vi "DHE_DO_INIT.vi"(8 "error in":errorcluster) -> (0 "error out":errorcluster, 2 "response":string)   [LabVIEW 2016]
uses:
  SDSU_GBLVariables.vi
panel:
  out "ControllerConfigCluster":T1
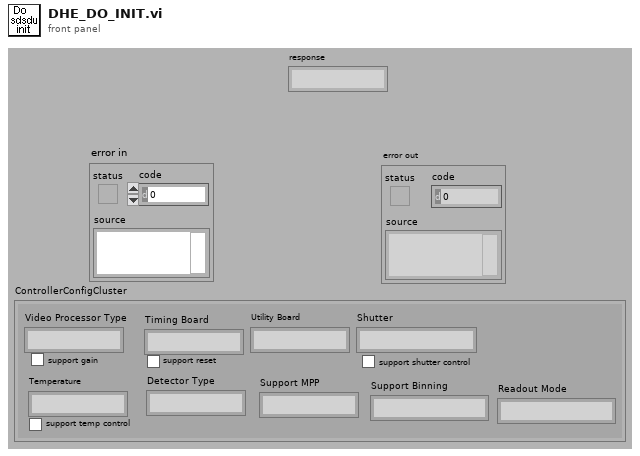
[diagram p1: front panel]
types:
  T1 = cluster{"Video Processor Type":string, "support gain":bool, "Timing Board":string, "support reset":bool, "Utility Board":string, "Shutter":string, "Temperature":string, "support temp control":bool, "Detector Type":string, "Support MPP":string, "Support Binning":string, "Readout Mode":string, "support shutter control":bool}
  T2 = enum16{"set all", "set", "get all", "get list", "get"}
  T3 = enum16{"READ FROM FILE", "GET ALL", "FIND BY NAME", "SET FIELD VALUE", "CLEAN"}
  T4 = enum16{"read from file", "find", "set", "set_to_default", "get all"}
  T5 = typedef "DatabaseHand_RefNum.ctl" = refnum<vi>
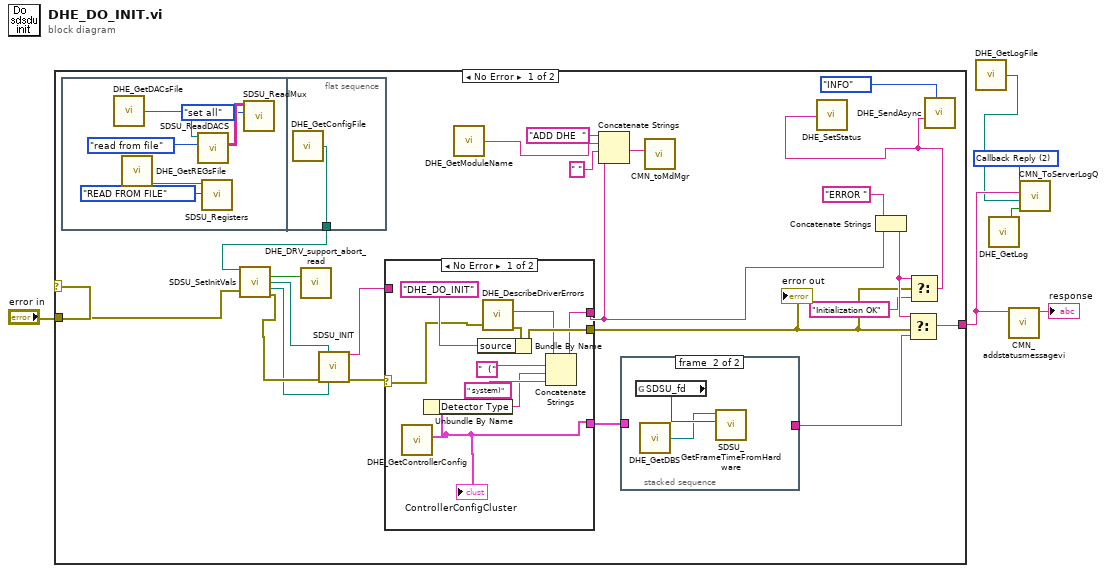
[diagram p0: block diagram]
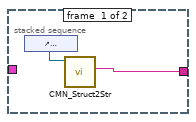
[diagram p2: hidden frame]
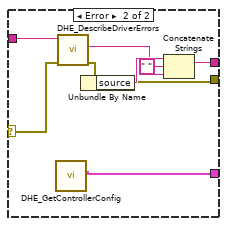
[diagram p3: hidden frame]
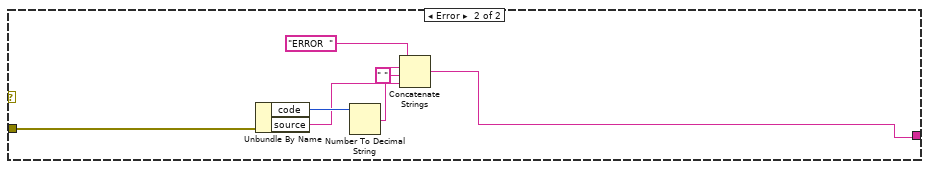
[diagram p4: hidden frame]
diagram:
  w5 = u16 2 items=["command", "imediateReply", "Callback Reply", "Information"] ("type")
  n1 = case shown="No Error" "error in" {
    tunnel: [w27 w62] -> w4
    tunnel: "error in" -> [w26 w64]
    frame No Error {
      n2 = flat-sequence {
        tunnel: [w35] -> w10
        frame #0 {
          n3 = call "DHE_GetDACsFile.vi"() -> ("DHE_DACFile"=w34:path)  [unwired: 9 out]
          n4 = call "DHE_GetREGsFile.vi"() -> ("DHE_REGsFile"=w32:path)  [unwired: 9 out]
          n5 = call "SDSU_ReadDACS.vi"("action"=T4."read from file", "file path"=w34) -> ("Table"=w30:string[][])  [unwired: 3 in, 6 out]
          n6 = call "SDSU_Registers.vi"("action"=T3."READ FROM FILE", "file path"=w32) -> ()  [unwired: 2 in, 8 out]
          n7 = call "SDSU_ReadMux.vi"("action"=T2."set all", "DACS"=w30) -> ()  [unwired: 3 in, 7 out]
        }
        frame #1 {
          n8 = call "DHE_GetConfigFile.vi"() -> ("DHE_ConfigFile"=w35:path)  [unwired: 9 out]
        }
      }
      n9 = call "SDSU_SetInitVals.vi"("ConfigPath"=w10, "error in"=w26) -> ("supabort"=w11:bool, "libdir out"=w8:path, "cmdtrans out"=w7:path, "error out"=w25:errorcluster)  [unwired: 10 out]
      n10 = call "DHE_DRV_support_abort_read.vi"("support abort?"=w11) -> ()  [unwired: 1 in, 14 out]
      n11 = call "SDSU_INIT.vi"("libdir"=w8, "error in"=w25, "cmdtrans"=w7) -> ("ImmedReplyString"=w9:string, "error out"=w24:errorcluster)  [unwired: 4 in, 7 out]
      n12 = case shown="No Error" w24 {
        selector: w24 -> [w42 w53]
        tunnel: [w43 w54] -> w18
        tunnel: [w48 w52] -> w16
        tunnel: [w41 w51] -> w14
        tunnel: w9 -> [_ w50]
        frame No Error {
          n13 = call "DHE_GetControllerConfig.vi"() -> ("ControllerConfigCluster"=w41:T1)  [unwired: 11 out]
          "ControllerConfigCluster" <- w41
          n14 = Unbundle By Name(w41) -> ("Detector Type"=w40:string)
          n15 = call "DHE_DescribeDriverErrors.vi"("error in (no error)"=w42) -> ("astroerrors"=w44:string, "error out"=w49:errorcluster)  [unwired: 2 in, 6 out]
          n16 = Bundle By Name(cluster=w49, "source"="DHE_DO_INIT") -> (w48:errorcluster)
          n17 = Concatenate Strings(w44, "  (", w40, " system)") -> (w43:string)
        }
        frame Error {
          n18 = call "DHE_GetControllerConfig.vi"() -> ("ControllerConfigCluster"=w51:T1)  [unwired: 11 out]
          n19 = call "DHE_DescribeDriverErrors.vi"("message"=w50, "error in (no error)"=w53) -> ("astroerrors"=w56:string, "error out"=w52:errorcluster)  [unwired: 1 in, 6 out]
          n20 = Unbundle By Name(w52) -> ("source"=w57:string)
          n21 = Concatenate Strings(w57, " " ("string"), w56) -> (w54:string)
        }
      }
      "error out" <- w16
      n22 = call "DHE_GetModuleName.vi"() -> ("DHE_ModuleName"=w12:string)  [unwired: 9 out]
      n23 = Concatenate Strings("ADD DHE  " ("string"), w12, " " ("string"), w18) -> (w19:string)
      n24 = stacked-sequence {
        tunnel: [w37 _] -> w21
        tunnel: w14 -> [_ _]
        frame #0 {
          n25 = control-ref of="ControllerConfigCluster"() -> (w36:refnum<vi>)
          n26 = call "CMN_Struct2Str.vi"("Cluster Ref"=w36) -> ("Controls Text"=w37:string)  [unwired: 2 in, 7 out]
        }
        frame #1 {
          n27 = global read "SDSU_GBLVariables.vi" "SDSU_fd"() -> (w39:i32)
          n28 = call "DHE_GetDBS.vi"() -> ("DHE_DBSRef"=w38:T5)  [unwired: 9 out]
          n29 = call "SDSU_GetFrameTimeFromHardware.vi"("fd"=w39, "Database Ref"=w38) -> ()  [unwired: 1 in, 9 out]
        }
      }
      n30 = call "CMN_toMdMgr.vi"("command"=w19) -> ()  [unwired: 10 out]
      n31 = Concatenate Strings("ERROR ", w18) -> (w23:string)
      n32 = Select(t=w23, s=w16, f=w21) -> (s? t:f=w27:string)
      n33 = Select(t=w23, s=w16, f="Initialization OK") -> (s? t:f=w13:string)
      n34 = call "DHE_SetStatus.vi"("DHE_Status"=w13) -> ()  [unwired: 9 out]
      n35 = call "DHE_SendAsync.vi"("type"=enum16{"ERROR", "WARNING", "INFO", "CHANGED"}."INFO", "Message"=w13) -> ()  [unwired: 2 in, 8 out]
    }
    frame Error {
      n36 = Unbundle By Name(w64) -> ("code"=w61:i32, "source"=w58:string)
      n37 = Number To Decimal String(number=w61) -> (decimal integer string=w60:string)  [unwired: 1 out]
      n38 = Concatenate Strings("ERROR  ", w60, " " ("Substring"), w58) -> (w62:string)
    }
  }
  n39 = call "DHE_GetLogFile.vi"() -> ("DHE_LogFile"=w3:path)  [unwired: 9 out]
  n40 = call "DHE_GetLog.vi"() -> ("DHE_log"=w2:bool)  [unwired: 9 out]
  n41 = call "CMN_addstatusmessagevi.vi"("message  in"=w4) -> ("message out"=→"response":string)  [unwired: 1 in, 9 out]
  n42 = call "CMN_ToServerLogQ.vi"("Log"=w2, "file"=w3, "string"=w4, "type"=w5) -> ()  [unwired: 2 in, 5 out]
